vi "LVProjectShortcut_RunEdit.vi"(8 "error in (no error)":errorcluster, 11 "Object":T1) -> (0 "error out":errorcluster)   [LabVIEW 2017, in "LVProject Shortcut.lvlib"]
doc: "Calls the Edit VI."
uses:
  LVProject Shortcut.lvlib
  <resource>/Framework/Providers/API/ItemRef.ctl
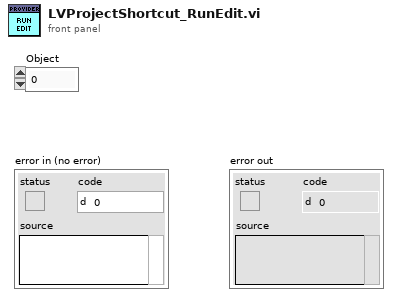
[diagram p1: front panel]
types:
  T1 = typedef "ItemRef.ctl" = u64
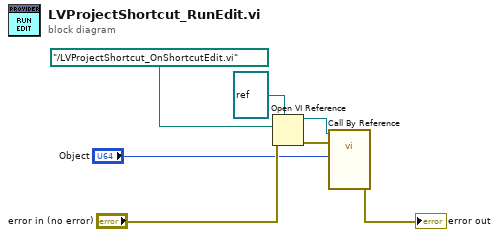
[diagram p0: block diagram]
diagram:
  n1 = Open VI Reference(type specifier VI Refnum (for type only)=refnum<vi> refnum, vi path=path "../LVProjectShortcut_OnShortcutEdit.vi", error in (no error)="error in (no error)") -> (vi reference=w3:refnum<vi>, error out=w2:errorcluster)  [unwired: 3 in]
  n2 = call-by-ref "?"(reference=w3, error in=w2, "Wizard"="Object") -> (error out=→"error out":errorcluster)  [unwired: 8 in, 2 out]
